vi "HAMULEC ON.vi"(10 "identifier":u32=1, 11 "Hamulec ON":bool) -> (3 "Message Cluster":T1)   [LabVIEW 2015]
uses:
  PC/QMH Fundamentals - Message Cluster.ctl
  CANFrameControl.ctl
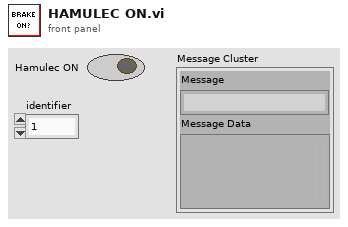
[diagram p1: front panel]
types:
  T1 = typedef "QMH Fundamentals - Message Cluster.ctl" = cluster{"Message":string, "Message Data":variant}
  T2 = typedef "CANFrameControl.ctl" = cluster{"identifier":u32, "extended?":bool, "type":u8, "payload":u8[]}
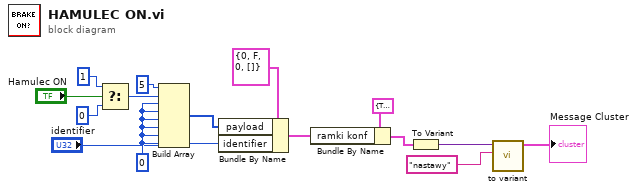
[diagram p0: block diagram]
diagram:
  w13 = u8 0 ("identifier")
  n1 = Select(t=u8 1 ("identifier"), s="Hamulec ON", f=u8 0 ("identifier")) -> (s? t:f=w11:u8)
  n2 = Build Array(u8 5 ("identifier"), w11, w13, w13, w13, w13, w13, w13) -> (w7:u8[])
  n3 = Bundle By Name(cluster=T2 {"identifier"=0, "extended?"=FALSE, "type"=0, "payload"=[]} ("CAN frame 2"), "payload"=w7, "identifier"="identifier") -> (w3:T2)
  n4 = Bundle By Name(cluster=cluster{"bool":bool, "ramki konf":T2} {"bool"=TRUE, "ramki konf"={"identifier"=0, "extended?"=TRUE, "type"=1, "payload"=[]}} ("jazda"), "ramki konf"=w3) -> (w4:cluster{"bool":bool, "ramki konf":T2})
  n5 = To Variant(anything=w4) -> (Variant=w2:variant)
  n6 = call "to variant.vi"("Message"="nastawy", "Variant"=w2) -> ("Message Cluster"=→"Message Cluster":T1)  [unwired: 9 in]
